vi "convertVideo.vi"(8 "error in (no error)":errorcluster, 9 "format":string, 10 "fileName":string, 11 "VideoConversionFacade in":refnum<class "VideoConversionFacade.lvclass">) -> (0 "error out":errorcluster, 2 "result out":refnum<class "VideoFile.lvclass">, 3 "VideoConversionFacade out":refnum<class "VideoConversionFacade.lvclass">)   [LabVIEW 2018, in "VideoConversionFacade.lvclass"]
uses:
  VideoConversionFacade.lvclass
  VideoFile Class/VideoFile.lvclass
  CodecFactory Class/CodecFactory.lvclass
  BitrateReader Class/BitrateReader.lvclass
  AudioMixer Class/AudioMixer.lvclass
  ConsoleOut/Print Options.ctl
  OggCompressionCodec Class/OggCompressionCodec.lvclass
  C:/Users/fflores/Documents/LabVIEW-Open-Projects/LabIVEW OOP Design Patterns/Facade Pattern/Codec Class/Codec.lvclass
  MPEG4CompressionCodec Class/MPEG4CompressionCodec.lvclass
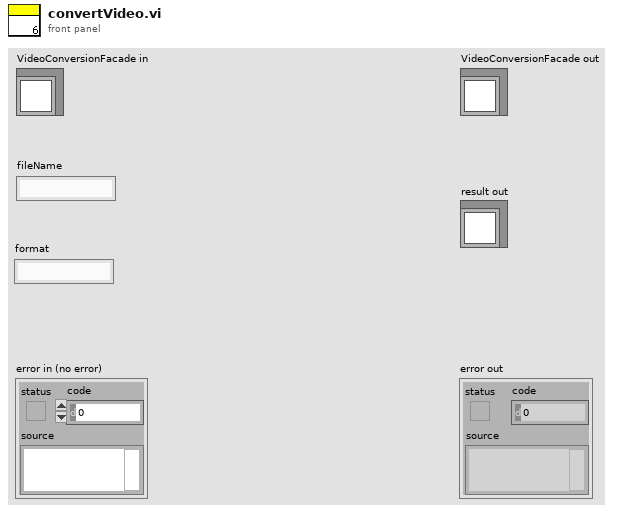
[diagram p1: front panel]
types:
  T1 = typedef "Print Options.ctl" = enum16{"Create", "Get Reference", "Print", "Print Header", "Close"}
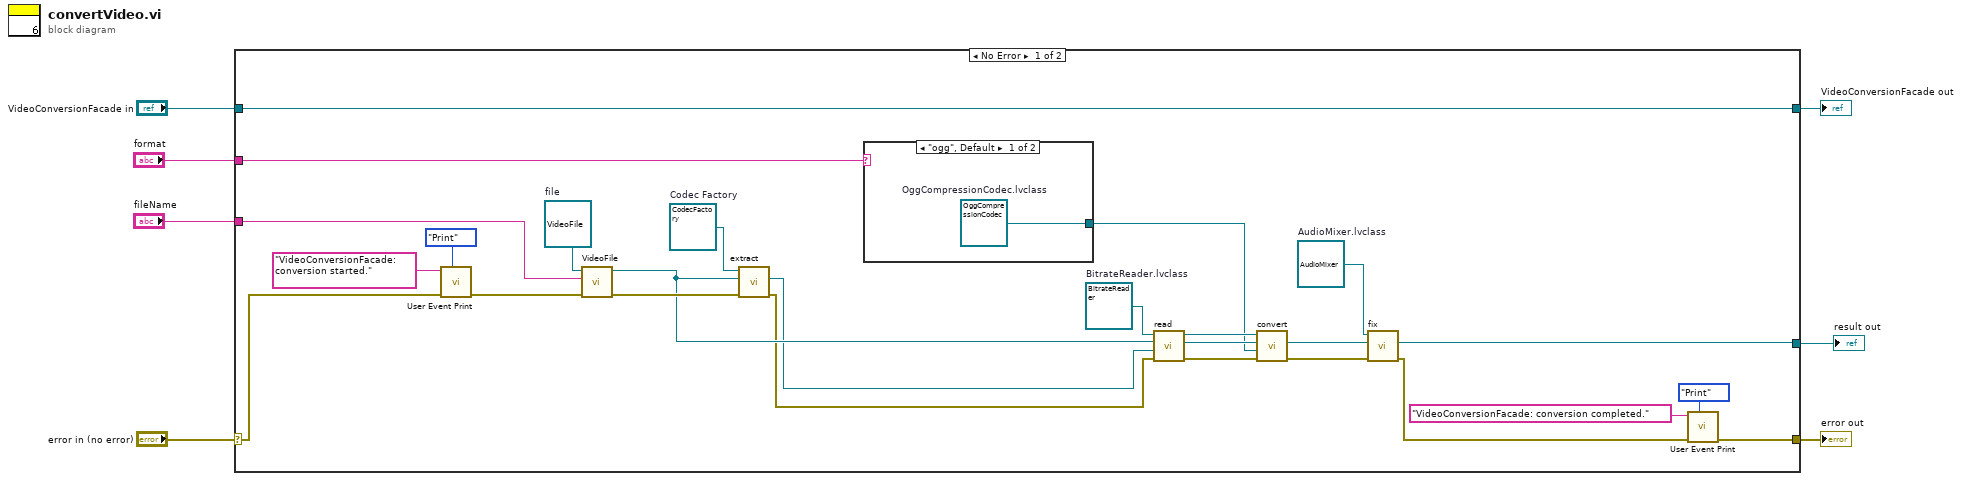
[diagram p0: block diagram]
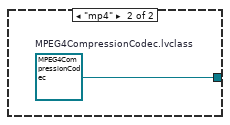
[diagram p2: hidden frame]
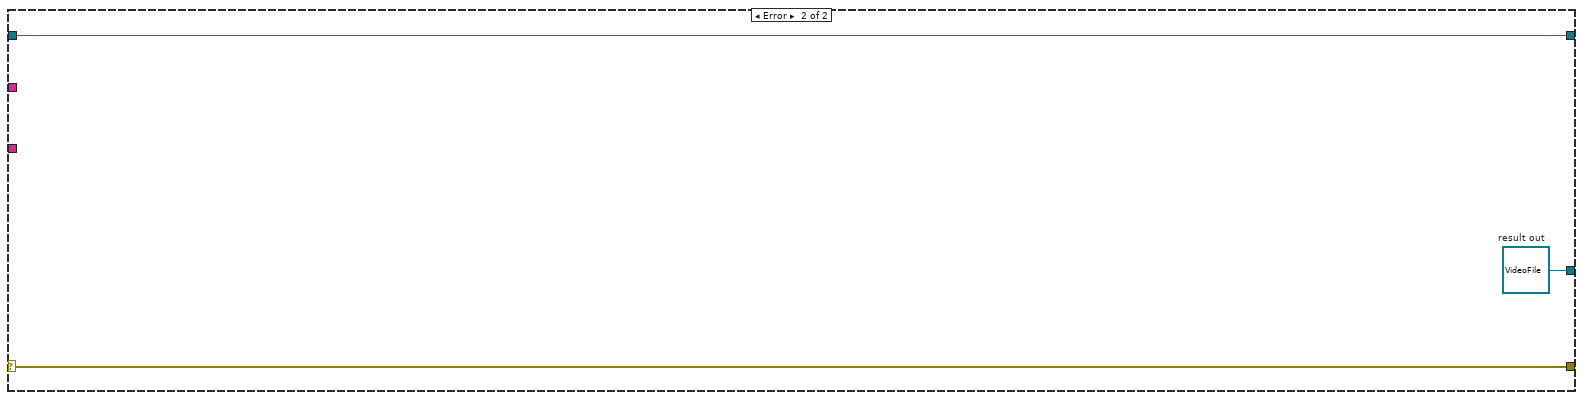
[diagram p3: hidden frame]
diagram:
  n1 = case shown="No Error" "error in (no error)" {
    selector: "error in (no error)" -> [w10 w38]
    tunnel: [w8 w38] -> w6
    tunnel: [w33 w37] -> w4
    tunnel: "VideoConversionFacade in" -> [w33 w37]
    tunnel: "fileName" -> [w21 _]
    tunnel: "format" -> [w29 _]
    tunnel: [w20 w36] -> w1
    frame No Error {
      w22 = refnum<class "AudioMixer.lvclass"> refnum  # AudioMixer.lvclass
      w27 = refnum<class "BitrateReader.lvclass"> refnum  # BitrateReader.lvclass
      w31 = refnum<class "CodecFactory.lvclass"> refnum  # Codec Factory
      w32 = refnum<class "VideoFile.lvclass"> refnum  # file
      n2 = call "User Event Print.vi"("Options"=Print_Options."Print", "error in (no error)"=w10, "String to Print"="VideoConversionFacade: conversion started." ("message")) -> ("error out"=w19:errorcluster)  [unwired: 7 in, 1 out]
      n3 = call "VideoFile.vi"("error in (no error)"=w19, "name"=w21, "VideoFile in"=w32) -> ("error out"=w30:errorcluster, "VideoFile out"=w28:refnum<class "VideoFile.lvclass">)  [unwired: 7 in]
      n4 = call "extract.vi"("error in (no error)"=w30, "VideoFile"=w28, "CodecFactory in"=w31) -> ("error out"=w13:errorcluster, "Codec"=w14:refnum<class "Codec.lvclass">)  [unwired: 6 in, 1 out]
      n5 = case shown="\"ogg\", Default" w29 {
        tunnel: [w34 w35] -> w24
        frame "ogg", Default {
          w34 = refnum<class "OggCompressionCodec.lvclass"> refnum  # OggCompressionCodec.lvclass
        }
        frame "mp4" {
          w35 = refnum<class "MPEG4CompressionCodec.lvclass"> refnum  # MPEG4CompressionCodec.lvclass
        }
      }
      n6 = call "read.vi"("error in (no error)"=w13, "Codec"=w14, "file"=w28, "BitrateReader in"=w27) -> ("error out"=w12:errorcluster, "VideoFile Out"=w25:refnum<class "VideoFile.lvclass">, "BitrateReader out"=w26:refnum<class "BitrateReader.lvclass">)  [unwired: 5 in]
      n7 = call "convert.vi"("error in (no error)"=w12, "Codec"=w24, "buffer"=w25, "BitrateReader in"=w26) -> ("error out"=w11:errorcluster, "buffer out"=w23:refnum<class "VideoFile.lvclass">)  [unwired: 5 in, 1 out]
      n8 = call "fix.vi"("error in (no error)"=w11, "result"=w23, "AudioMixer in"=w22) -> ("error out"=w9:errorcluster, "result out"=w20:refnum<class "VideoFile.lvclass">)  [unwired: 6 in, 1 out]
      n9 = call "User Event Print.vi"("Options"=Print_Options."Print", "error in (no error)"=w9, "String to Print"="VideoConversionFacade: conversion completed." ("message")) -> ("error out"=w8:errorcluster)  [unwired: 7 in, 1 out]
    }
    frame Error {
      w36 = refnum<class "VideoFile.lvclass"> refnum  # result out
    }
  }
  "error out" <- w6
  "VideoConversionFacade out" <- w4
  "result out" <- w1
